vi "RichToFlatnixnet_grpc_DbUndeployRequest.vi"(5 "OutputClusterType":T1, 11 "InputCluster":T2) -> (3 "OutputCluster":T1)   [LabVIEW 2025, in "grpc-xnet_client.lvlib"]
uses:
  grpc-xnet_client.lvlib
  nixnet_grpc_DbUndeployRequest.ctl
  nixnet_grpc_DbUndeployRequest_Flat.ctl
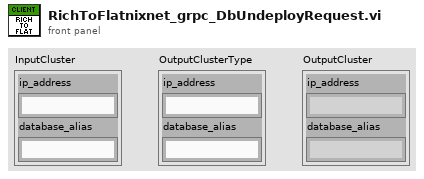
[diagram p1: front panel]
types:
  T1 = typedef "grpc-xnet_client.lvlib/nixnet_grpc_DbUndeployRequest_Flat.ctl" = cluster{"ip_address":string, "database_alias":string}
  T2 = typedef "grpc-xnet_client.lvlib/nixnet_grpc_DbUndeployRequest.ctl" = cluster{"ip_address":string, "database_alias":string}
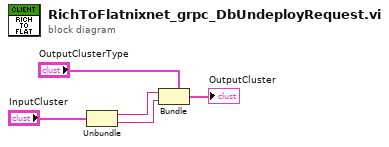
[diagram p0: block diagram]
diagram:
  n1 = Unbundle "Unbundle"("InputCluster") -> ("ip_address"=w2:string, "database_alias"=w1:string)
  n2 = Bundle "Bundle"(cluster="OutputClusterType", "ip_address"=w2, "database_alias"=w1) -> (→"OutputCluster":T1)
